vi "ingresarDatosEquipos.vi"(8 "error in (no error)":errorcluster, 11 "Calibrador in":refnum<class "Calibrador.lvclass">) -> (0 "error out":errorcluster, 3 "Calibrador out":refnum<class "Calibrador.lvclass">)   [LabVIEW 2019, in "Calibrador.lvclass"]
uses:
  Calibrador.lvclass
  Calibrador.lvclass/Calibrador.ctl
  QMH/Message Queue/Enqueue Message (Single).vi
  <vilib>/Utility/error.llb/Error Cluster From Error Code.vi
  RerenceAllControlsToolkit/_get control reference by name.vi
  RerenceAllControlsToolkit/_get mutiple control reference by name.vi
  <vilib>/ErrorRing/Error Ring.xnode
  QMH/Message Queue/Message Queue.lvlib
  QMH/User Event - Stop/User Event - Stop.lvlib
panel:
  in  "guardar":bool
  out "Resultado":string
  in  "Direccion":string
  in  "Nombre":string
  in  "salir":bool
  in  "cb_clase_equipo":string(combo)
  out "estandar":string
  in  "cb_modelo":string(combo)
  in  "numero_serial_equipo":string
  out "equipoSeleccionado":string
  in  "cb_marca_equipo":string(combo)
  # "Equipo"
  # "Cliente"
  # "Dirección"
  # "Nombre"
  # "Clase"
  # "Estándar"
  # "Modelo"
  # "Número Serial"
  # "Marca"
  # "Equipo"
  # "Ingreso Datos de Instrumentos y Accesorios"
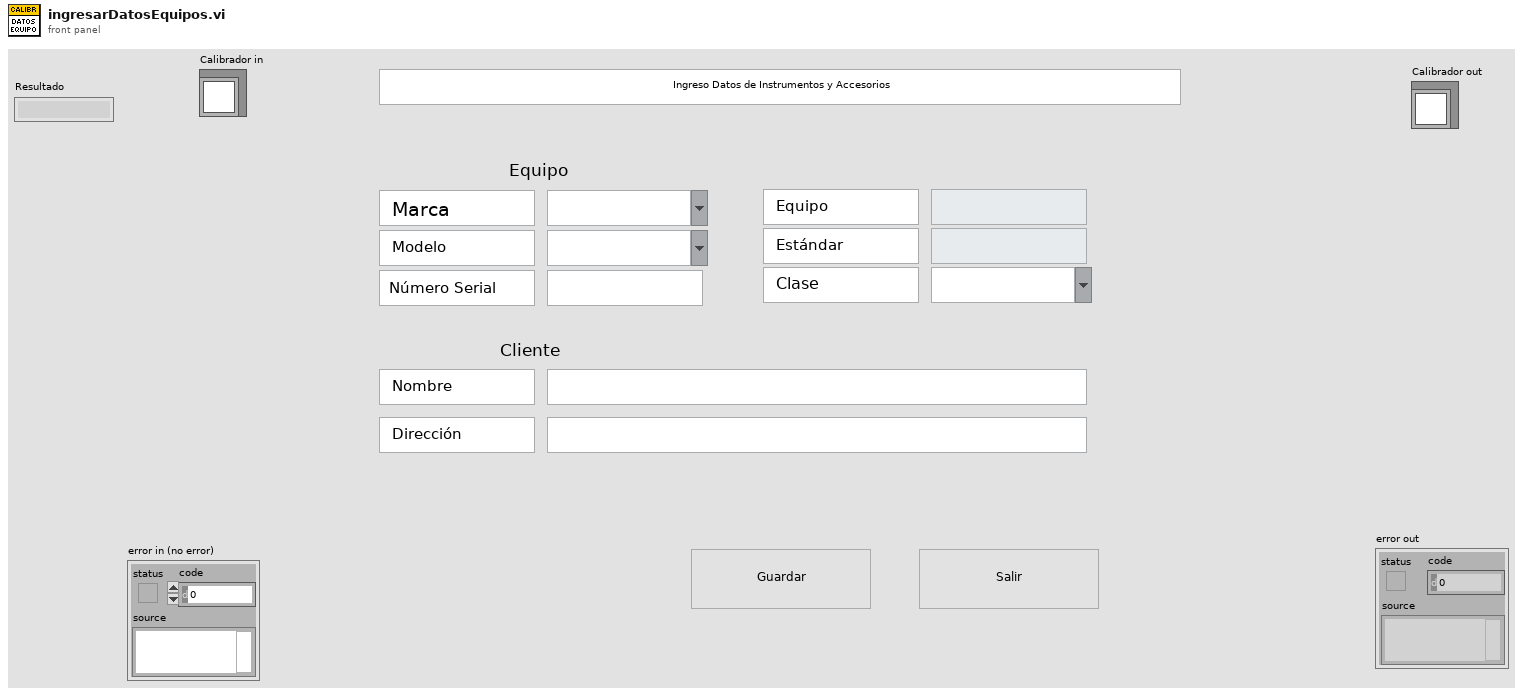
[diagram p1: front panel]
types:
  T1 = typedef "Message Queue.lvlib/All Message Queues.ctl" = cluster{"MHL":refnum<queue>, "Inst_CNT90":refnum<queue>, "Inst_DS360":refnum<queue>, "Inst_Keithley2002":refnum<queue>, "Inst_DAQ":refnum<queue>, "BD":refnum<queue>, "Pistofono":refnum<queue>, "Nexus":refnum<queue>}
  T2 = cluster{"ControlName":string, "ControlReference":refnum<vi>}[]
  T3 = cluster{string, "Control references":cluster{"ControlName":string, "ControlReference":refnum<vi>}[]}
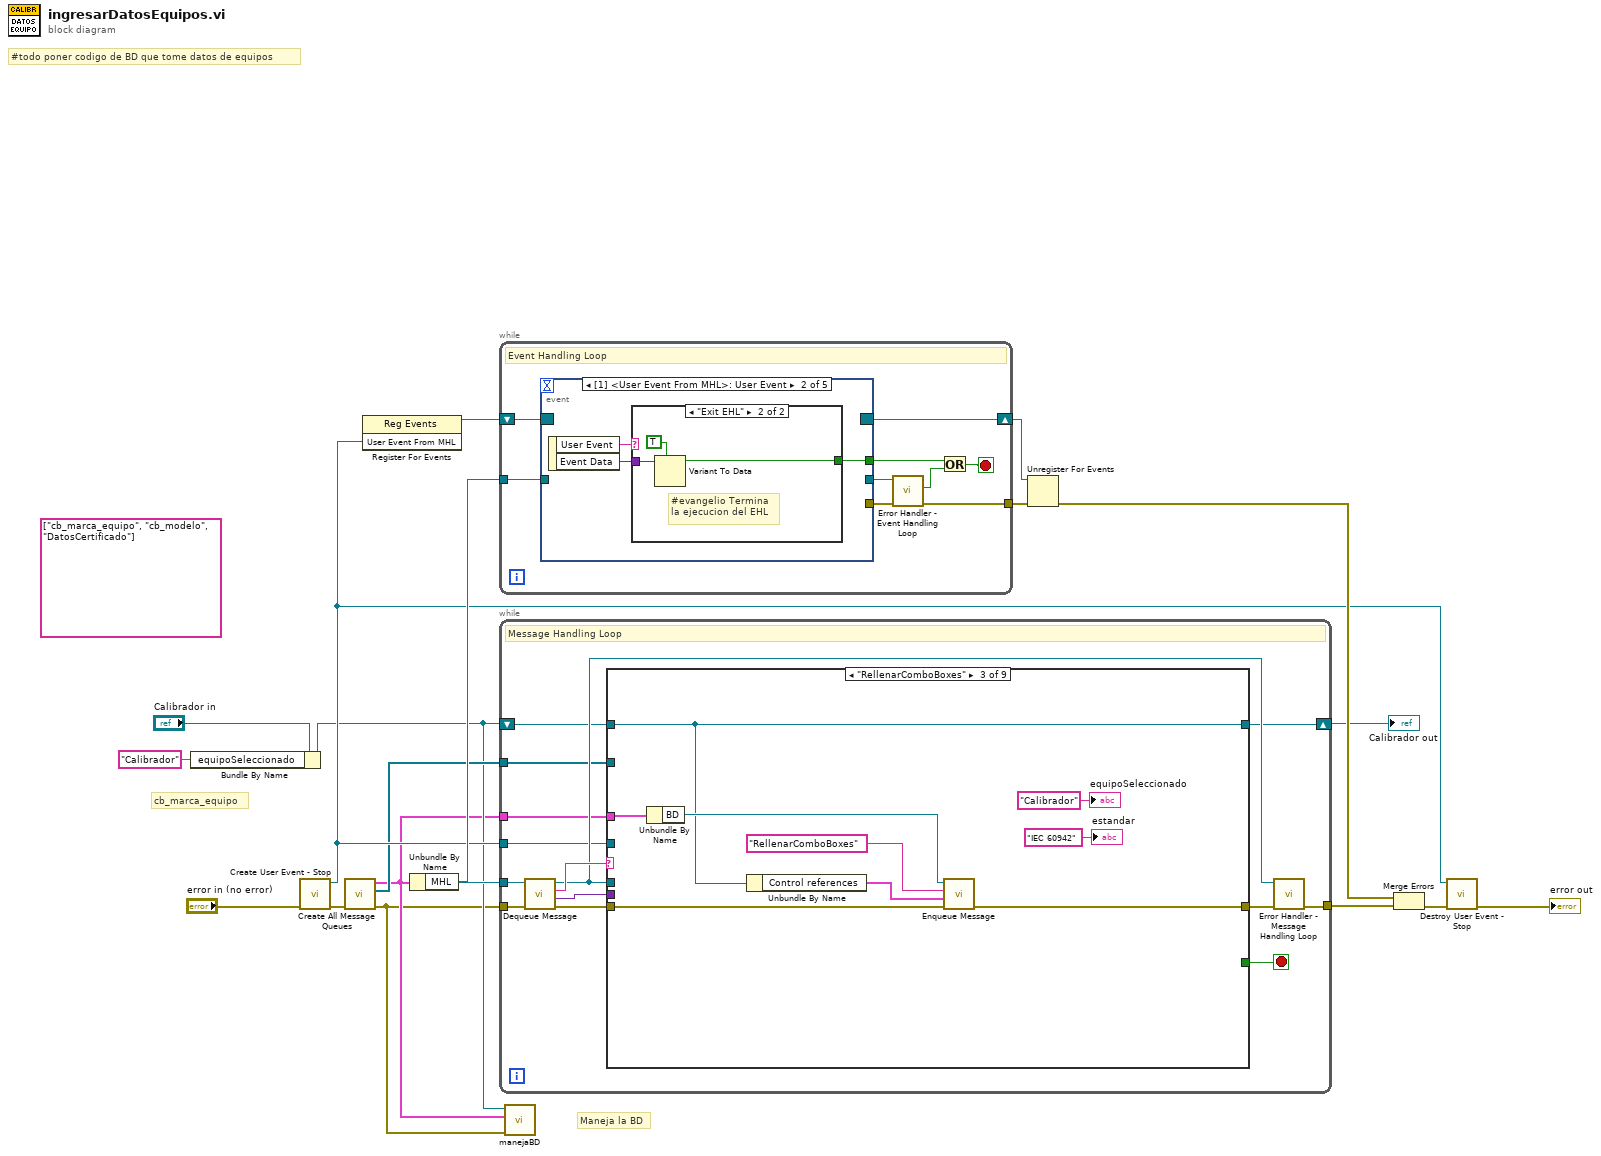
[diagram p0: block diagram]
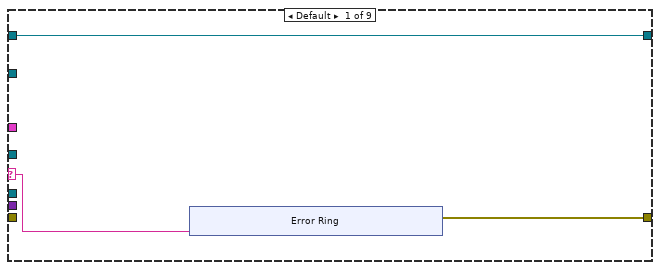
[diagram p2: hidden frame]
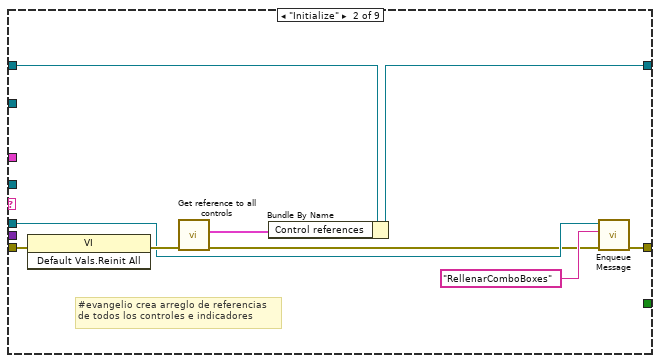
[diagram p3: hidden frame]
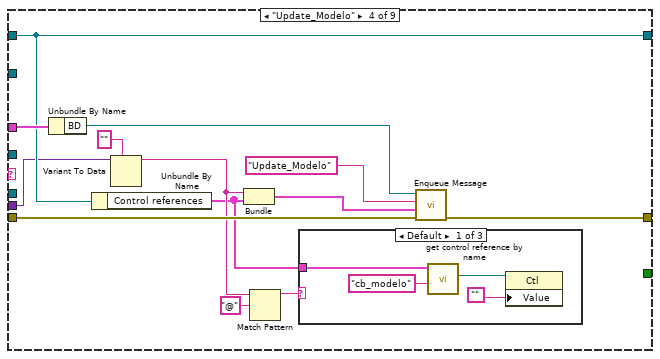
[diagram p4: hidden frame]
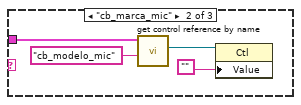
[diagram p5: hidden frame]
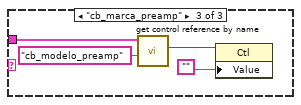
[diagram p6: hidden frame]
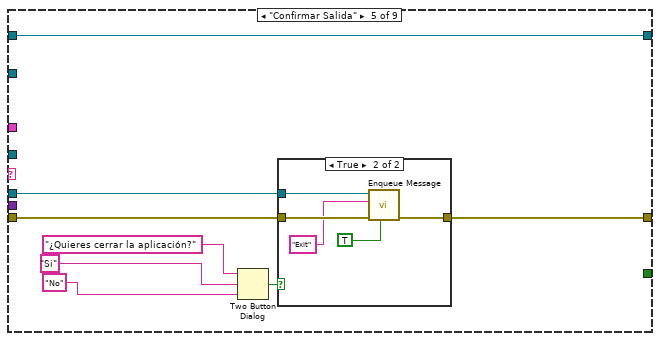
[diagram p7: hidden frame]
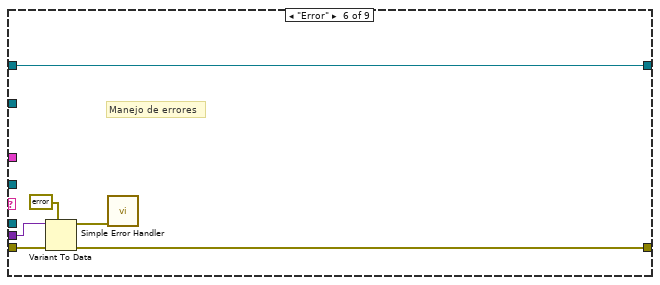
[diagram p9: hidden frame]
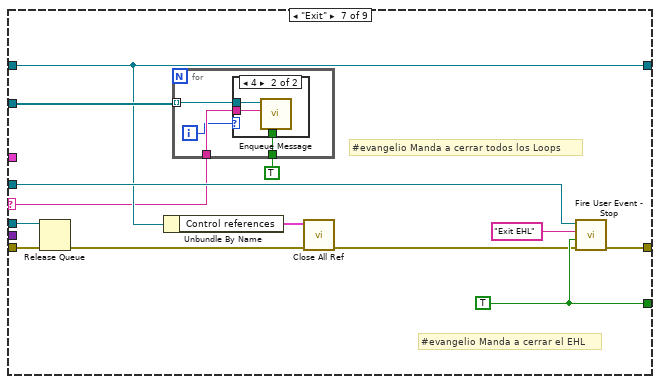
[diagram p10: hidden frame]
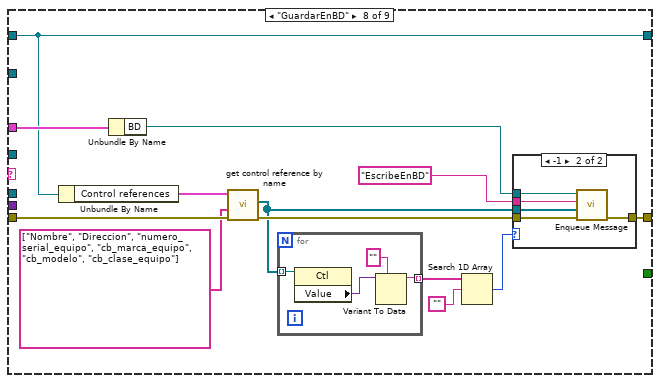
[diagram p12: hidden frame]
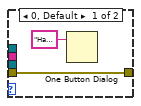
[diagram p13: hidden frame]
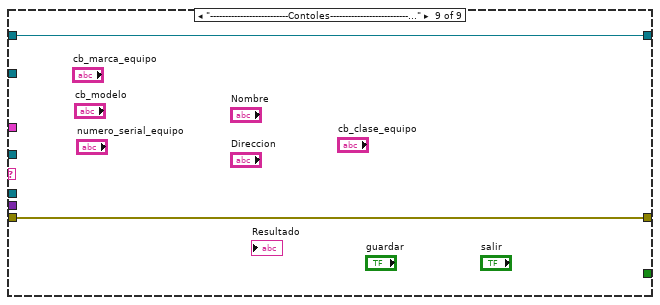
[diagram p14: hidden frame]
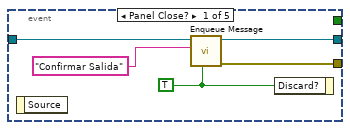
[diagram p15: hidden frame]
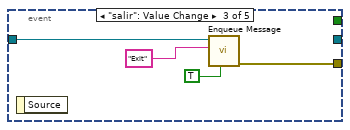
[diagram p17: hidden frame]
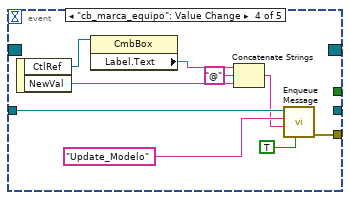
[diagram p18: hidden frame]
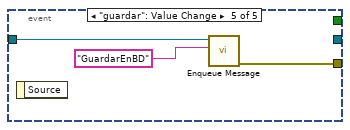
[diagram p19: hidden frame]
diagram:
  (unwired) string[] ["cb_marca_equipo", "cb_modelo", "DatosCertificado"]
  # "#todo poner codigo de BD que tome datos de equipos"
  # "cb_marca_equipo"
  # "Maneja la BD"
  n1 = Bundle By Name(cluster="Calibrador in", "equipoSeleccionado"="Calibrador") -> (w5:refnum<class "Calibrador.lvclass">)
  n2 = call "Create User Event - Stop.vi"("error in (no error)"="error in (no error)") -> ("error out"=w15:errorcluster, "User Event From MHL"=w10:refnum<user-event>)  [unwired: 9 in]
  n3 = call "Create All Message Queues.vi"("error in (no error)"=w15) -> ("error out"=w3:errorcluster, "PL Queues Array"=w9:refnum<queue>[], "All Message Queues out"=w4:T1)  [unwired: 8 in]
  n4 = register-events(w10) -> (reference out=w18:refnum<event-registration>)  [unwired: 2 in, 1 out]
  n5 = Unbundle By Name(w4) -> ("MHL"=w14:refnum<queue>)
  n6 = while {
    tunnel: w14 -> [w27]
    tunnel: [w23] -> w17
    shift-right: [w25] -> w16
    shift-left: w18 -> [w26]
    stop <- w19 stop-if-true
    # "Event Handling Loop"
    n7 = event shown="[1] <User Event From MHL>: User Event" {
      selector: w26 -> [_ _ _ _ _]
      dyn-events: [_ _ _ _ _] -> w25
      timeout: _ -> [_ _ _ _ _]
      tunnel: w27 -> [w30 _ w41 w50 w53]
      tunnel: [w32 _ w42 w51 w54] -> w24
      tunnel: [w31 _ _ _ _] -> w22
      tunnel: [_ w33 _ _ _] -> w20
      event Panel Close? {
        w28 = TRUE
        n8 = event-data() -> ()  [unwired: 1 in, 1 out]
        n9 = call-poly "Enqueue Message.vi"("Priority Message? (F)"=w28, "Message"="Confirmar Salida", "Message Queue"=w30) -> ("error out"=w32:errorcluster, "dup Message Queue"=w31:refnum<queue>)  [unwired: 7 in]
        n10 = event-data("Discard?"=w28) -> ()  [unwired: 1 in, 1 out]
      }
      event User Event {
        n11 = event-data() -> ("User Event"=w35:string, "Event Data"=w34:variant)  [unwired: 1 in]
        n12 = case shown="\"Exit EHL\"" w35 {
          tunnel: w34 -> [_ w37]
          tunnel: [_ w36] -> w33
          frame Default {
          }
          frame "Exit EHL" {
            # "#evangelio Termina\nla ejecucion del EHL"
            n13 = Variant To Data(type=TRUE, Variant=w37) -> (data=w36:bool)  [unwired: 1 in, 1 out]
          }
        }
      }
      event "salir": Value Change {
        n14 = event-data() -> ()  [unwired: 1 in, 1 out]
        n15 = call-poly "Enqueue Message.vi"("Priority Message? (F)"=TRUE, "Message"="Exit", "Message Queue"=w41) -> ("error out"=w42:errorcluster)  [unwired: 7 in, 1 out]
      }
      event "cb_marca_equipo": Value Change {
        n16 = event-data() -> ("CtlRef"=w47:refnum<vi>, "NewVal"=w46:string)  [unwired: 1 in]
        n17 = property class="CmbBox"(reference=w47) -> ("Label.Text"=w44:string)  [unwired: 1 in, 2 out]
        n18 = Concatenate Strings(w44, "@" ("string"), w46) -> (w45:string)
        n19 = call-poly "Enqueue Message.vi"("Priority Message? (F)"=TRUE, "Message Data"=w45, "Message"="Update_Modelo", "Message Queue"=w50) -> ("error out"=w51:errorcluster)  [unwired: 6 in, 1 out]
      }
      event "guardar": Value Change {
        n20 = event-data() -> ()  [unwired: 1 in, 1 out]
        n21 = call-poly "Enqueue Message.vi"("Message"="GuardarEnBD", "Message Queue"=w53) -> ("error out"=w54:errorcluster)  [unwired: 8 in, 1 out]
      }
    }
    n22 = call "Error Handler - Event Handling Loop.vi"("error in (no error)"=w24, "Message Queue"=w22) -> ("dup error in"=w23:errorcluster, "Error?"=w21:bool)  [unwired: 7 in, 1 out]
    n23 = Or(x=w20, y=w21) -> (x .or. y?=w19:bool)
  }
  n24 = while {
    tunnel: w3 -> [w68]
    tunnel: w14 -> [w67]
    tunnel: [w61] -> w12
    shift-right: [w59] -> w6
    shift-left: w5 -> [w60]
    tunnel: w4 -> [w57]
    tunnel: w10 -> [w56]
    tunnel: w9 -> [w55]
    stop <- w58 stop-if-true
    # "Message Handling Loop"
    n25 = call "Dequeue Message.vi"("error in (no error)"=w68, "Message Queue"=w67) -> ("error out"=w64:errorcluster, "Message Data"=w65:variant, "Message"=w66:string, "dup Message Queue"=w63:refnum<queue>)  [unwired: 6 in]
    n26 = case shown="\"RellenarComboBoxes\"" w66 {
      selector: w66 -> [w70 _ _ _ _ _ w144 _ _]
      tunnel: w63 -> [_ w84 _ _ w122 _ w154 _ _]
      tunnel: w65 -> [_ _ _ w103 _ w137 _ _ _]
      tunnel: w64 -> [_ w87 w96 w109 w128 w138 w153 w171 w187]
      tunnel: [w69 w85 w95 w108 w127 w139 w152 w166 w187] -> w62
      tunnel: w60 -> [w71 w80 w91 w104 w129 w141 w145 w168 w186]
      tunnel: [w71 w82 w91 w104 w129 w141 w145 w168 w186] -> w59
      tunnel: [_ _ _ _ _ _ w149 _ _] -> w58
      tunnel: w57 -> [_ _ w93 w106 _ _ _ w174 _]
      tunnel: w56 -> [_ _ _ _ _ _ w151 _ _]
      tunnel: w55 -> [_ _ _ _ _ _ w146 _ _]
      frame Default {
        n27 = xnode "Error Ring"("parameter 0"=w70) -> ("error out"=w69:errorcluster)
      }
      frame "Initialize" {
        # "#evangelio crea arreglo de referencias\nde todos los controles e indicadores"
        n28 = invoke class="VI" method="Default Vals.Reinit All"(error in=w87) -> (error out=w86:errorcluster)  [unwired: 2 in, 2 out]
        n29 = call "Get reference to all controls.vi"("error in (no error)"=w86) -> ("error out"=w79:errorcluster, "Control references"=w81:T2)  [unwired: 5 in]
        n30 = Bundle By Name(cluster=w80, "Control references"=w81) -> (w82:refnum<class "Calibrador.lvclass">)
        n31 = call-poly "Enqueue Message.vi"("error in (no error)"=w79, "Message"="RellenarComboBoxes", "Message Queue"=w84) -> ("error out"=w85:errorcluster)  [unwired: 7 in, 1 out]
      }
      frame "RellenarComboBoxes" {
        n32 = Unbundle By Name(w93) -> ("BD"=w92:refnum<queue>)
        n33 = Unbundle By Name(w91) -> ("Control references"=w90:T2)
        n34 = call-poly "Enqueue Message.vi"("error in (no error)"=w96, "Message Data"=w90, "Message"="RellenarComboBoxes", "Message Queue"=w92) -> ("error out"=w95:errorcluster)  [unwired: 6 in, 1 out]
        "equipoSeleccionado" <- "Calibrador" ("equipoSeleccionado")
        "estandar" <- "IEC 60942" ("estandar")
      }
      frame "Update_Modelo" {
        n35 = Unbundle By Name(w106) -> ("BD"=w105:refnum<queue>)
        n36 = Unbundle By Name(w104) -> ("Control references"=w97:T2)
        n37 = Variant To Data(type="", Variant=w103) -> (data=w100:string)  [unwired: 1 in, 1 out]
        n38 = Bundle(w100, "Control references"=w97) -> (w101:T3)  [unwired: 1 in]
        n39 = Match Pattern(string=w100, regular expression="@") -> (before substring=w98:string)  [unwired: 1 in, 3 out]
        n40 = case shown="Default" w98 {
          tunnel: w97 -> [w110 w114 w118]
          frame Default {
            n41 = call-poly "get control reference by name.vi"("Control name"="cb_modelo", "Control references"=w110) -> ("Ctl Refnum"=w111:refnum<vi>)  [unwired: 4 in, 1 out]
            n42 = property class="Ctl"(reference=w111, "Value"="") -> ()  [unwired: 1 in, 2 out]
          }
          frame "cb_marca_mic" {
            n43 = call-poly "get control reference by name.vi"("Control name"="cb_modelo_mic", "Control references"=w114) -> ("Ctl Refnum"=w115:refnum<vi>)  [unwired: 4 in, 1 out]
            n44 = property class="Ctl"(reference=w115, "Value"="") -> ()  [unwired: 1 in, 2 out]
          }
          frame "cb_marca_preamp" {
            n45 = call-poly "get control reference by name.vi"("Control name"="cb_modelo_preamp", "Control references"=w118) -> ("Ctl Refnum"=w119:refnum<vi>)  [unwired: 4 in, 1 out]
            n46 = property class="Ctl"(reference=w119, "Value"="") -> ()  [unwired: 1 in, 2 out]
          }
        }
        n47 = call-poly "Enqueue Message.vi"("error in (no error)"=w109, "Message Data"=w101, "Message"="Update_Modelo", "Message Queue"=w105) -> ("error out"=w108:errorcluster)  [unwired: 6 in, 1 out]
      }
      frame "Confirmar Salida" {
        n48 = Two Button Dialog(message="¿Quieres cerrar la aplicación?", 1:"No" ("T button name (\"OK\")"), 2:"Si" ("T button name (\"OK\")")) -> (T button?=w123:bool)
        n49 = case shown="True" w123 {
          tunnel: w128 -> [w130 w135]
          tunnel: [w130 w134] -> w127
          tunnel: w122 -> [_ w133]
          frame False {
          }
          frame True {
            n50 = call-poly "Enqueue Message.vi"("Priority Message? (F)"=TRUE, "error in (no error)"=w135, "Message"="Exit", "Message Queue"=w133) -> ("error out"=w134:errorcluster)  [unwired: 6 in, 1 out]
          }
        }
      }
      frame "Error" {
        # "Manejo de errores"
        n51 = Variant To Data(error in=w138, type=errorcluster {"status"=FALSE, "code"=0, "source"=""} ("error constant"), Variant=w137) -> (data=w136:errorcluster, error out=w139:errorcluster)
        n52 = call <vilib>:"Simple Error Handler.vi"("error in (no error)"=w136) -> ()  [unwired: 4 in, 5 out]
      }
      frame "Exit" {
        w149 = TRUE
        # "#evangelio Manda a cerrar todos los Loops"
        # "#evangelio Manda a cerrar el EHL"
        n53 = Release Queue(queue=w154, error in (no error)=w153) -> (error out=w143:errorcluster)  [unwired: 1 in, 2 out]
        n54 = Unbundle By Name(w145) -> ("Control references"=w148:T2)
        n55 = for {
          tunnel: w146 -> [w158] mode=indexing
          tunnel: w144 -> [w157]
          tunnel: TRUE -> [w156]
          i -> [w155]
          n56 = case shown="4" w155 {
            tunnel: w158 -> [_ w161]
            tunnel: w157 -> [_ w160]
            tunnel: w156 -> [_ w159]
            frame Default {
            }
            frame 4 {
              n57 = call-poly "Enqueue Message.vi"("Priority Message? (F)"=w159, "Message"=w160, "Message Queue"=w161) -> ()  [unwired: 7 in, 2 out]
            }
          }
        }
        n58 = call "Close All Ref.vi"("error in (no error)"=w143, "Control references"=w148) -> ("error out"=w142:errorcluster)  [unwired: 9 in]
        n59 = call "Fire User Event - Stop.vi"("error in (no error)"=w142, "Event Data"=w149, "User Event"="Exit EHL", "User Event in"=w151) -> ("error out"=w152:errorcluster)  [unwired: 7 in]
      }
      frame "GuardarEnBD" {
        n60 = Unbundle By Name(w168) -> ("Control references"=w169:T2)
        n61 = Unbundle By Name(w174) -> ("BD"=w173:refnum<queue>)
        n62 = call-poly "get control reference by name.vi"("error in (no error)"=w171, "Control names"=string[] ["Nombre", "Direccion", "numero_serial_equipo", "cb_marca_equipo", "cb_modelo", "cb_clase_equipo"], "Control references"=w169) -> ("error out"=w170:errorcluster, "References"=w165:refnum<vi>[])  [unwired: 3 in]
        n63 = for {
          tunnel: w165 -> [w185] mode=indexing
          tunnel: [w183] -> w164 mode=indexing
          n64 = property class="Ctl"(reference=w185) -> ("Value"=w184:variant)  [unwired: 1 in, 2 out]
          n65 = Variant To Data(type="", Variant=w184) -> (data=w183:string)  [unwired: 1 in, 1 out]
        }
        n66 = Search 1D Array(1D array=w164, element="") -> (index of element=w162:i32)  [unwired: 1 in]
        n67 = case shown="-1" w162 {
          tunnel: w173 -> [_ w181]
          tunnel: "EscribeEnBD" ("Message") -> [_ w180]
          tunnel: w170 -> [w176 w179]
          tunnel: [w176 w178] -> w166
          tunnel: w165 -> [_ w177]
          frame 0, Default {
            n68 = One Button Dialog(message="Hay campos vacios") -> ()  [unwired: 1 in, 1 out]
          }
          frame -1 {
            n69 = call-poly "Enqueue Message.vi"("error in (no error)"=w179, "Message Data"=w177, "Message"=w180, "Message Queue"=w181) -> ("error out"=w178:errorcluster)  [unwired: 6 in, 1 out]
          }
        }
      }
      frame "--------------------------Contoles---------------------------" {
      }
    }
    n70 = call "Error Handler - Message Handling Loop.vi"("error in (no error)"=w62, "Message Queue"=w63) -> ("dup error in"=w61:errorcluster)  [unwired: 8 in, 1 out]
  }
  "Calibrador out" <- w6
  n71 = call "manejaBD.vi"("error in"=w3, "All Message Queues in"=w4, "Calibrador in"=w5) -> ()  [unwired: 8 in, 1 out]
  n72 = Unregister For Events(event registration refnum=w16, error in=w17) -> (error out=w13:errorcluster)
  n73 = Merge Errors(w13, w12) -> (w11:errorcluster)
  n74 = call "Destroy User Event - Stop.vi"("error in (no error)"=w11, "User Event"=w10) -> ("error out"=→"error out":errorcluster)  [unwired: 9 in]
